vi "Check Special Tags.vi"(0 "source":string) -> (1 "Before Tag (source)":string, 2 "After Tag (special data)":string, 3 "Tag Found?":T1)   [LabVIEW 2020]
uses:
  TagReturnType.ctl
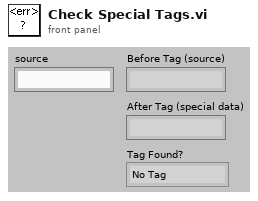
[diagram p1: front panel]
types:
  T1 = typedef "TagReturnType.ctl" = enum16{"No Tag", "<err>", "<append>"}
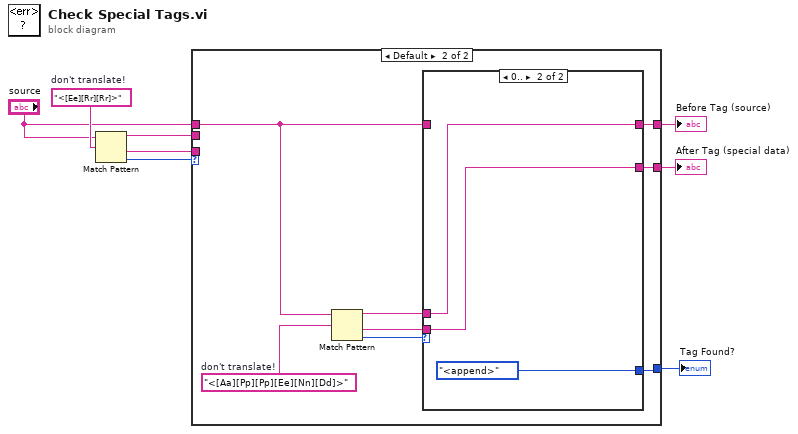
[diagram p0: block diagram]
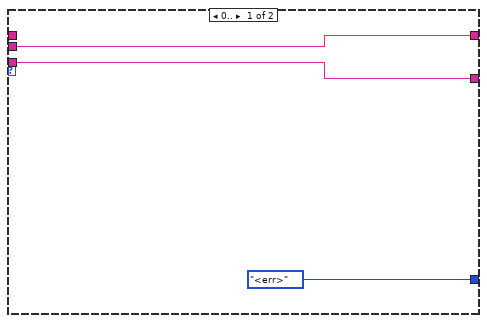
[diagram p2: hidden frame]
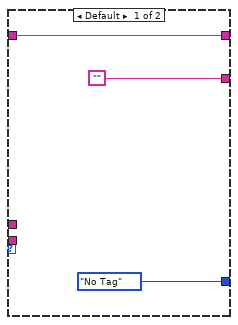
[diagram p3: hidden frame]
diagram:
  w8 = "<[Ee][Rr][Rr]>"  # don't translate!
  n1 = Match Pattern(string="source", regular expression=w8) -> (before substring=w7:string, after substring=w6:string, offset past match=w1:i32)  [unwired: 1 in, 1 out]
  n2 = case shown="Default" w1 {
    tunnel: w7 -> [w10 _]
    tunnel: w6 -> [w11 _]
    tunnel: [w11 w17] -> w5
    tunnel: [w10 w15] -> w4
    tunnel: [TagReturnType."<err>" ("Tag Found?") w14] -> w3
    tunnel: "source" -> [_ w13]
    frame 0.. {
    }
    frame Default {
      w19 = "<[Aa][Pp][Pp][Ee][Nn][Dd]>"  # don't translate!
      n3 = Match Pattern(string=w13, regular expression=w19) -> (before substring=w18:string, after substring=w16:string, offset past match=w12:i32)  [unwired: 1 in, 1 out]
      n4 = case shown="0.." w12 {
        tunnel: w18 -> [_ w24]
        tunnel: ["" w25] -> w17
        tunnel: w16 -> [_ w25]
        tunnel: [w22 w24] -> w15
        tunnel: [TagReturnType."No Tag" ("Tag Found?") TagReturnType."<append>" ("Tag Found?")] -> w14
        tunnel: w13 -> [w22 _]
        frame Default {
        }
        frame 0.. {
        }
      }
    }
  }
  "After Tag (special data)" <- w5
  "Before Tag (source)" <- w4
  "Tag Found?" <- w3
